vi "LockedHeading.vi"(7 "LockHeading":bool, 9 "Heading In":dbl) -> (3 "LockedHeading":dbl)   [LabVIEW 2017]
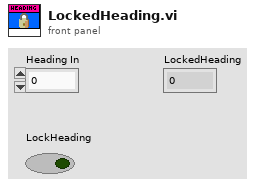
[diagram p1: front panel]
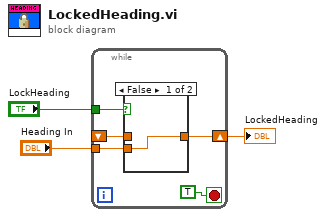
[diagram p0: block diagram]
diagram:
  n1 = while {
    tunnel: "LockHeading" -> [w7]
    tunnel: "Heading In" -> [w6]
    shift-right: [w5] -> w3
    shift-left: _ -> [w4]
    stop <- TRUE stop-if-true
    n2 = case shown="False" w7 {
      tunnel: w6 -> [w9 _]
      tunnel: [w9 w10] -> w5
      tunnel: w4 -> [_ w10]
      frame False {
      }
      frame True {
      }
    }
  }
  "LockedHeading" <- w3
